vi "Agilent SNA Read Trigger Mode.vi"(6 "Channel":i8=1 min=1 max=99 step=1, 7 "Agilent SNA & SWP":T1, 8 "error in (no error)":errorcluster, 11 "VISA Resource Names":T3) -> (0 "error out":errorcluster, 2 "Trigger Mode":T2, 3 "dup VISA Resource Names":T3)   [LabVIEW 2011]
doc: "This VI for the HP8753B Network Analyzers reads the stimulus values. Except when performing log sweeps and freq list sweeps, this VI uses the start and stop values and the number of points to calcuate the stimulus values."
uses:
  TypeDefs/Agilent SNA VISA.ctl
  TypeDefs/Agilent SNA Trigger Mode.ctl
  TypeDefs/Agilent SNA Instrument Info.ctl
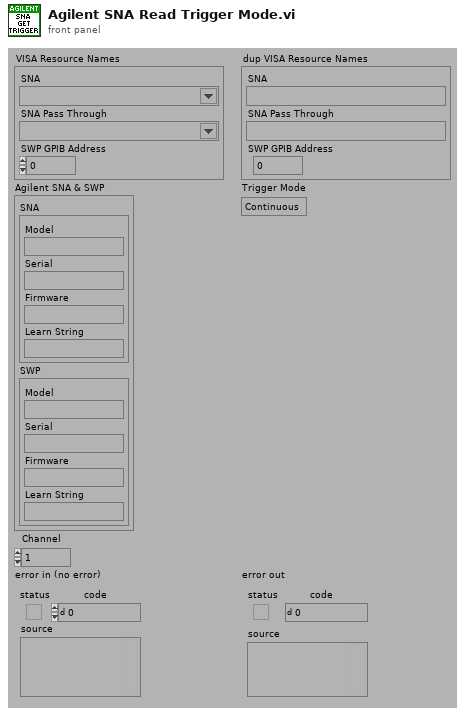
[diagram p1: front panel]
types:
  T1 = typedef "Agilent SNA Instrument Info.ctl" = cluster{"SNA":cluster{"Model":string, "Serial":string, "Firmware":string, "Learn String":string}, "SWP":cluster{"Model":string, "Serial":string, "Firmware":string, "Learn String":string}}
  T2 = typedef "Agilent SNA Trigger Mode.ctl" = enum16{"Continuous", "Hold", "Single"}
  T3 = typedef "Agilent SNA VISA.ctl" = cluster{"SNA":refnum<visa-resource-name>, "SNA Pass Through":refnum<visa-resource-name>, "SWP GPIB Address":i32}
  T4 = typedef "Agilent SNA Model.ctl" = enum16{"Not Supported", "8757X"}
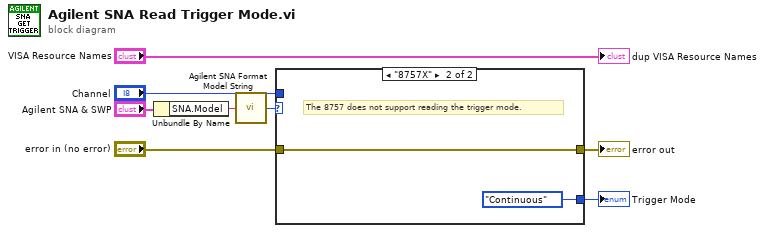
[diagram p0: block diagram]
diagram:
  n1 = Unbundle By Name("Agilent SNA & SWP") -> ("SNA.Model"=w2:string)
  n2 = call "Agilent SNA Format Model String.vi"("Model String"=w2) -> ("Model"=w5:T4)
  n3 = case shown="\"8757X\"" w5 {
    tunnel: "error in (no error)" -> [w9 w10]
    tunnel: [w9 w10] -> w7
    tunnel: [_ Agilent_SNA_Trigger_Mode."Continuous"] -> w6
    tunnel: "Channel" -> [_ _]
    frame "Not Supported" {
    }
    frame "8757X" {
      # "The 8757 does not support reading the trigger mode."
    }
  }
  "error out" <- w7
  "Trigger Mode" <- w6
  "dup VISA Resource Names" <- "VISA Resource Names"
